vi "high_level_file_io.vi"() -> ()   [LabVIEW 2018]
uses:
  <vilib>/Utility/file.llb/Write Delimited Spreadsheet (DBL).vi
panel:
  out "웨이브폼 차트":dbl(graph)
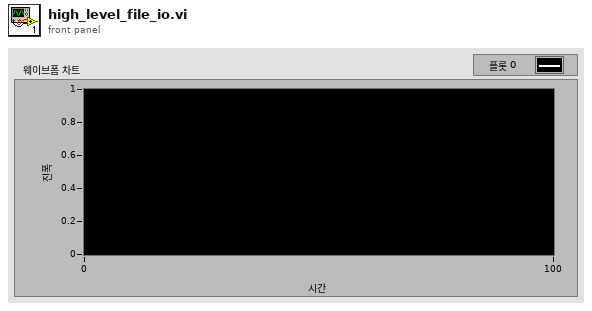
[diagram p1: front panel]
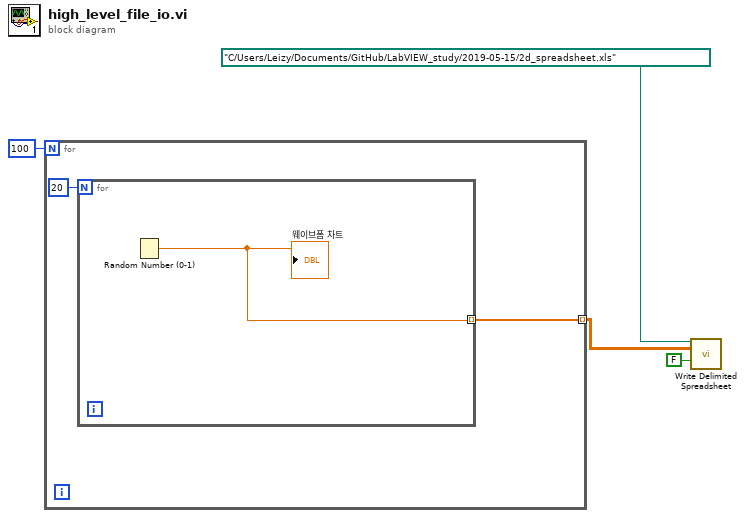
[diagram p0: block diagram]
diagram:
  n1 = for {
    N: 100 -> [_]
    tunnel: [w6] -> w3 mode=indexing
    n2 = for {
      N: 20 -> [_]
      tunnel: [w7] -> w6 mode=indexing
      n3 = Random Number (0-1)() -> (number: 0 to 1=w7:dbl)
      "웨이브폼 차트" <- w7
    }
  }
  n4 = call-poly <vilib>:"Write Delimited Spreadsheet.vi"("file path (dialog if empty)"=path "C:/Users/Leizy/Documents/GitHub/LabVIEW_study/2019-05-15/2d_spreadsheet.xls", "2D data"=w3, "append to file? (new file:F)"=FALSE) -> ()  [unwired: 11 in, 2 out]
